vi "U8array2U32.vi"(8 "hi 2":u8, 9 "lo 2":u8, 10 "hi":u8, 11 "lo":u8) -> (3 "(hi.lo)":u32)   [LabVIEW 2020, in "AIM664LV.lvlib"]
uses:
  AIM664LV.lvlib
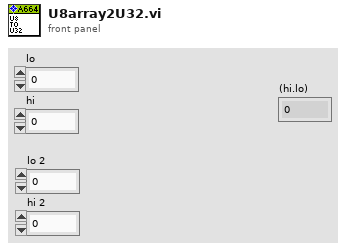
[diagram p1: front panel]
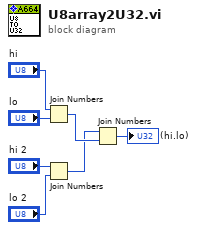
[diagram p0: block diagram]
diagram:
  n1 = Join Numbers(hi="hi", lo="lo") -> ((hi.lo)=w2:u16)
  n2 = Join Numbers(hi="hi 2", lo="lo 2") -> ((hi.lo)=w1:u16)
  n3 = Join Numbers(hi=w1, lo=w2) -> ((hi.lo)=→"(hi.lo)":u32)
